vi "Increment.vi"(8 "error in (no error)":errorcluster, 11 "Complex in":refnum<class "Complex.lvclass">) -> (0 "error out":errorcluster, 3 "Complex out":refnum<class "Complex.lvclass">)   [LabVIEW 2018, in "Complex.lvclass"]
uses:
  Complex.lvclass
  Complex.lvclass/Complex.ctl
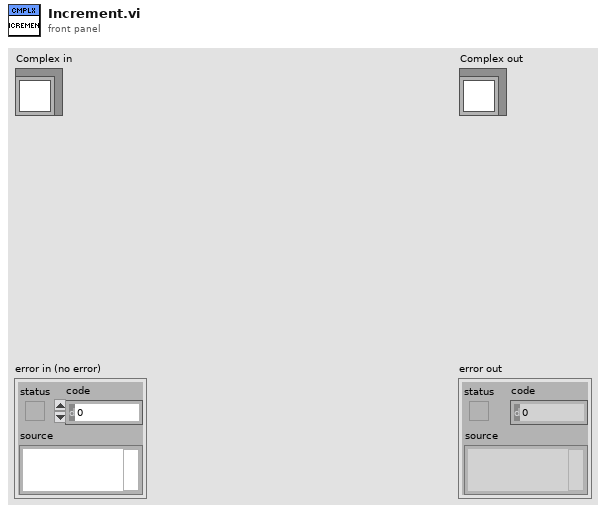
[diagram p1: front panel]
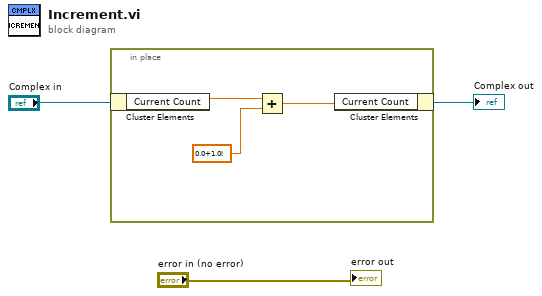
[diagram p0: block diagram]
diagram:
  n1 = in-place {
    n2 = in-place-cluster #1("Complex in") -> ("Current Count"=w6:cdb)
    n3 = Add(x=w6, y=cdb 0.0+1.0i) -> (x+y=w4:cdb)
    n4 = in-place-cluster #1("Current Count"=w4) -> (→"Complex out":refnum<class "Complex.lvclass">)
  }
  "error out" <- "error in (no error)"
